vi "HelloWorld.vi"() -> ()   [LabVIEW 2021]
panel:
  out "Output":string
  in  "Input":string
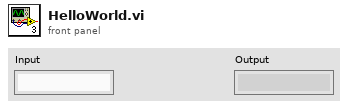
[diagram p1: front panel]
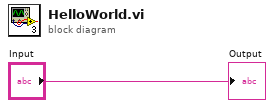
[diagram p0: block diagram]
diagram:
  "Output" <- "Input"
